vi "AFM_PI_control_trajTrack.vi"() -> ()   [LabVIEW 2017]
uses:
  controls/controlParams_tracktraj.ctl
  <vilib>/rvi/Emulation/niFpgaGetClockAttributes.vi
  <vilib>/rvi/Emulation/niFpgaSctlEmulationGetInTimedLoop.vi
  <vilib>/rvi/Emulation/niFpgaEmulationReportErrorSimple.vi
  <vilib>/rvi/eio/common/nirviEmuTemplateMethod_errors.vi
  <vilib>/rvi/Emulation/niFpgaCriticalErrorInLSC.vi
  <vilib>/rvi/DataTransferAndStorage/Container/Common/niFpgaContainerExecOnDevCompGetState.vi
  <vilib>/rvi/Emulation/niFpgaEmulationIsFPGAContextNoSignature.vi
  <vilib>/rvi/DataTransferAndStorage/Container/Common/niFpgaContainerGetUniqueNameForEmu.vi
  <vilib>/rvi/Memory/Memory_Emulation/niFpgaMemoryEmulationCacheClearOnFirstRun.vi
  <vilib>/rvi/Memory/Memory_Emulation/nirvimemoryEmulationManagerCache_MakeExclusive.vi
  <vilib>/rvi/Memory/Memory_Emulation/niFpgaMemoryEmulationValidateCache.vi
  <vilib>/rvi/Memory/Memory_Emulation/nirvimemoryEmulationManagerCache_InsertValue.vi
  <vilib>/Utility/error.llb/Clear Errors.vi
  <vilib>/rvi/Memory/Memory_Emulation/nirvimemoryEmulationManagerCache_ReleaseExclusive.vi
  <vilib>/rvi/Memory/Memory_Emulation/nirvimemoryEmulationManagerCache_GetValue.vi
  <vilib>/rvi/Memory/Memory_Emulation/nirvimemoryEmulationManagerCache_SetValue.vi
  <vilib>/rvi/Emulation/niFpgaProcessEmulError.vi
  <vilib>/rvi/interface/RandomDataEmulation/niFpgaRandomDataHandleErrors.vi
  <vilib>/eio/EIONode/EIONode.xnode
  <vilib>/rvi/DataTransferAndStorage/Container/XNode/niFpgaContainer.xnode
  <vilib>/rvi/DataTransferAndStorage/Register/Emulation/niFpgaRegisterEmulationRefIn.vi
  <vilib>/rvi/interface/RandomDataEmulation/nirviRandomDataFpgaReadWriteTemplate.vi
  <vilib>/rvi/FXPMathLib/FxpSub/XNode/nifxpmath_Sub.xnode
  <vilib>/rvi/FXPMathLib/sim/FxpSim.dll
panel:
  out "yk":sgl
  out "u_xk":sgl
  out "yuxk TO":bool
  out "YK TO":bool
  out "UK TO":bool
  in  "Cluster":T1={"umax"=3.0, "y_ref(k)"=0.0, "Ki"=0.0, "y(k) (from plant)"=0.0, "ND"=0, "NS"=0, "u_Kx_ref(k)"=0.0} {"u_Kx_ref(k)" format="%#_13g"; "Ki" format="%#_13g"; "y_ref(k)" format="%#_13g"; "umax" format="%#_13g"}
  out "Unstable Traj":bool
  out "Loop Done":bool
  in  "Settle Ticks":i16=1000
  in  "False  = cont run":bool=TRUE
  in  "Abort":bool=TRUE
  in  "iters":i16=1
  in  "ymax":sgl=4.0 format="%#_13g"
  in  "TsTicks":i16
  out "Loop Ticks (benchmark)":i16
  out "NS":i16=2
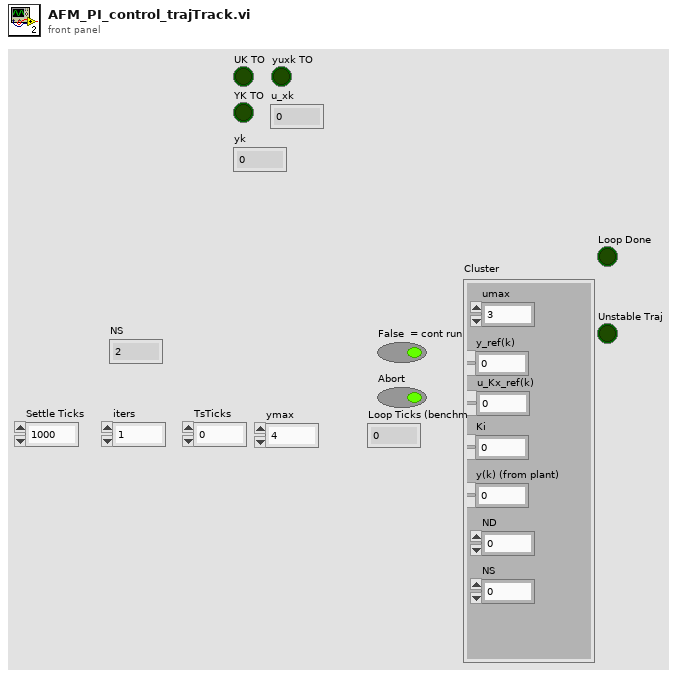
[diagram p1: front panel]
types:
  T1 = typedef "controlParams_tracktraj.ctl" = cluster{"umax":sgl, "y_ref(k)":sgl, "Ki":sgl, "y(k) (from plant)":sgl, "ND":i16, "NS":i16, "u_Kx_ref(k)":sgl}
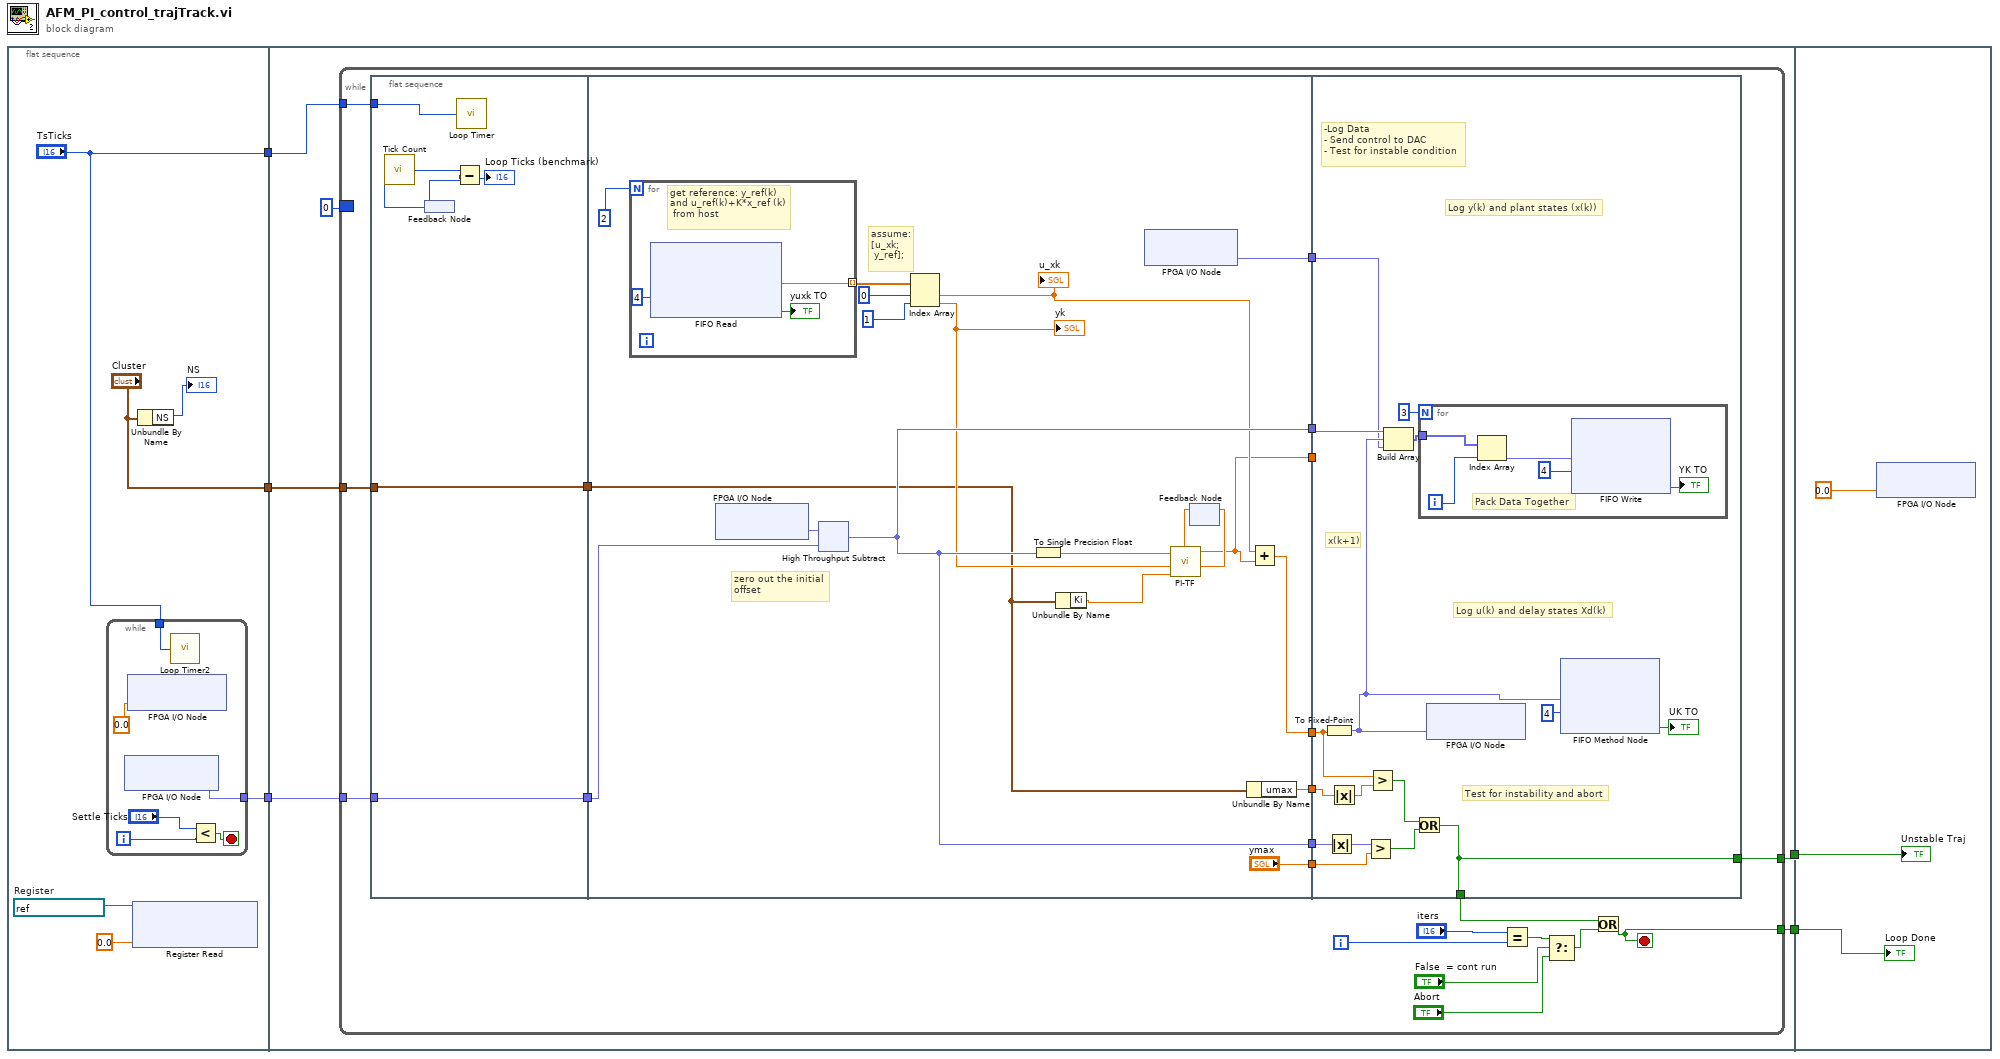
[diagram p0: block diagram]
diagram:
  n1 = flat-sequence {
    tunnel: ["TsTicks"] -> w5
    tunnel: [w11] -> w4
    tunnel: ["Cluster"] -> w2
    tunnel: w5 -> [w22]
    tunnel: w4 -> [w21]
    tunnel: [w20] -> w3
    tunnel: w2 -> [w19]
    tunnel: [w18] -> w1
    tunnel: w3 -> [w94]
    tunnel: w1 -> [w93]
    frame #0 {
      w9 = refnum<k21> "accumulator"  # Register
      # "Load Matrix Data"
      n2 = while {
        tunnel: [w17] -> w11
        tunnel: "TsTicks" -> [w16]
        i -> [w12]
        stop <- w14 stop-if-true
        n3 = xnode "FPGA I/O Node"() -> ("Mod2/AI0"=w17:fxp<+/-,24,5>)  [unwired: 1 in, 1 out]
        n4 = xnode "FPGA I/O Node"("Mod1/AO0"=sgl 0.0) -> ()  [unwired: 1 in, 1 out]
        n5 = call "Loop Timer2"("Count(Ticks)"=w16) -> ()  [unwired: 1 out]
        n6 = Less?(x="Settle Ticks", y=w12) -> (x < y?=w14:bool)
      }
      n7 = xnode ("Register Read")("Data"=sgl 0.0, "Register In"=w9) -> ()  [unwired: 1 out]
      n8 = Unbundle By Name("Cluster") -> ("NS"=→"NS":i16)
    }
    frame #1 {
      n9 = while {
        border: i16 0 -> [_]
        tunnel: w22 -> [w36]
        tunnel: w21 -> [w34]
        tunnel: [w32] -> w20
        tunnel: w19 -> [w30]
        tunnel: [w29] -> w18
        i -> [w41]
        stop <- w32 stop-if-true
        n10 = flat-sequence {
          tunnel: w36 -> [w47]
          tunnel: w34 -> [w46]
          tunnel: [w46] -> w33
          tunnel: [w45] -> w31
          tunnel: w30 -> [w45]
          tunnel: [w56] -> w44
          tunnel: [w62] -> w35
          tunnel: w33 -> [w68]
          tunnel: w31 -> [w53]
          tunnel: [w62] -> w28
          tunnel: [w61] -> w27
          tunnel: ["ymax"] -> w26
          tunnel: [w54] -> w25
          tunnel: [w51] -> w24
          tunnel: w44 -> [w81]
          tunnel: [w75] -> w43
          tunnel: w35 -> [w85]
          tunnel: [w75] -> w29
          tunnel: w28 -> [w84]
          tunnel: w27 -> [w80]
          tunnel: w26 -> [w78]
          tunnel: w25 -> [_]
          tunnel: w24 -> [w72]
          frame #0 {
            n11 = call "Tick Count"() -> ("Tick Count(Ticks)"=w48:u32)
            n12 = feedback #1() -> (w49:u32)
            n13 = feedback-in #1(w48) -> ()
            n14 = Subtract(x=w48, y=w49) -> (x-y=→"Loop Ticks (benchmark)":u32)
            n15 = call "Loop Timer"("Count(Ticks)"=w47) -> ()  [unwired: 1 out]
          }
          frame #1 {
            # "assume:\n[u_xk;\n y_ref];"
            # "zero out the initial \noffset"
            n16 = for {
              N: i16 2 -> [_]
              tunnel: [w70] -> w65 mode=indexing
              # "get reference: y_ref(k)\nand u_ref(k)+K*x_ref (k)\n from host"
              n17 = xnode ("FIFO Read")("Timeout"=i16 4) -> ("Element"=w70:sgl, "Timed Out?"=→"yuxk TO":bool)  [unwired: 1 in, 1 out]
            }
            n18 = xnode "FPGA I/O Node"() -> ("Mod2/AI0"=w67:fxp<+/-,24,5>)  [unwired: 1 in, 1 out]
            n19 = xnode "High Throughput Subtract"("x"=w67, "y"=w68) -> ("x-y"=w62:fxp<+/-,40,6>)
            n20 = Index Array(array=w65, index #1=i16 0, index #2=i16 1) -> (element #1=w57:sgl, element #2=w58:sgl)
            "u_xk" <- w57
            "yk" <- w58
            n21 = To Single Precision Float(number=w62) -> (single precision float=w59:sgl)
            n22 = Unbundle By Name(w53) -> ("Ki"=w52:sgl)
            n23 = xnode "FPGA I/O Node"() -> ("Mod2/AI1"=w51:fxp<+/-,24,5>)  [unwired: 1 in, 1 out]
            n24 = feedback #2() -> (w54:sgl)  [unwired: 1 in]
            n25 = call "PI-TF.vi"("u(k-1)"=w54, "Ki"=w52, "setpoint"=w58, "y(k)"=w59) -> ("u(k)"=w55:sgl)  [unwired: 7 in]
            n26 = feedback-in #2(w55) -> ()
            n27 = Unbundle By Name(w53) -> ("umax"=w61:sgl)
            n28 = Add(x=w57, y=w54) -> (x+y=w56:sgl)
          }
          frame #2 {
            # "x(k+1)"
            # "Log u(k) and delay states Xd(k)"
            # "Log y(k) and plant states (x(k))"
            # "-Log Data\n- Send control to DAC\n- Test for instable condition"
            # "Test for instability and abort"
            n29 = To Fixed-Point(number=w81) -> (fixed-point=w74:fxp<+/-,32,6>)  [unwired: 1 in]
            n30 = Absolute Value(x=w84) -> (abs(x)=w87:fxp<+,40,6>)
            n31 = Absolute Value(x=w80) -> (abs(x)=w79:sgl)
            n32 = Greater?(x=w87, y=w78) -> (0:w76:bool)
            n33 = Greater?(x=w81, y=w79) -> (0:w77:bool)
            n34 = Build Array(w85, w74, w72) -> (w86:fxp<+/-,40,6>[])
            n35 = Or(x=w77, y=w76) -> (x .or. y?=w75:bool)
            n36 = for {
              N: 3 -> [_]
              tunnel: w86 -> [w90]
              i -> [w91]
              # "Pack Data Together"
              n37 = Index Array(array=w90, index=w91) -> (element=w89:fxp<+/-,40,6>)
              n38 = xnode ("FIFO Write")("Element"=w89, "Timeout"=i16 4) -> ("Timed Out?"=→"YK TO":bool)  [unwired: 1 in, 1 out]
            }
            n39 = xnode "FPGA I/O Node"("Mod1/AO0"=w74) -> ()  [unwired: 1 in, 1 out]
            n40 = xnode ("FIFO Method Node")("Element"=w74, "Timeout"=i16 4) -> ("Timed Out?"=→"UK TO":bool)  [unwired: 1 in, 1 out]
          }
        }
        n41 = Equal?(x="iters", y=w41) -> (x = y?=w39:bool)
        n42 = Select(t=w39, s="False  = cont run", f="Abort") -> (s? t:f=w40:bool)
        n43 = Or(x=w43, y=w40) -> (x .or. y?=w32:bool)
      }
    }
    frame #2 {
      n44 = xnode "FPGA I/O Node"("Mod1/AO0"=sgl 0.0) -> ()  [unwired: 1 in, 1 out]
      "Loop Done" <- w94
      "Unstable Traj" <- w93
    }
  }
